vi "NI_9222_Anologue_DAQ3_FPGA_Host.vi"() -> ()   [LabVIEW 2013]
uses:
  <vilib>/userDefined/High Color/nirio_resource_hc.ctl
  <vilib>/rvi/interface/common/niFpgaWaitOnOcc.vi
  <vilib>/FPGAPlugInAG/cRIO-9068/niLvFpga_Open_cRIO-9068.vi
  <vilib>/rvi/interface/common/dynamic/niFpgaDynamicAddResources.vi
  <vilib>/Utility/error.llb/Error Cluster From Error Code.vi
  <vilib>/rvi/errors/niLvFpgaAdjustHostInterfaceError.vi
  <vilib>/RVI Host/nirviSupport.llb/nirviErrorClusterFromErrorCode.vi
  <vilib>/FPGAPlugInAG/Dynamic/niLvFpga_Close_Dynamic.vi
  <vilib>/rvi/interface/nirviOpenFPGA/nirviOpenFPGA.xnode
  FPGA Bitfiles/cRioProject1_FPGATarget_NI9222AnologueDA_7Q1sMVkmokY.lvbitx
  NI_9222_Anologue_DAQ2_FPGA.vi
  <vilib>/rvi/interface/nirviMethod/nirviMethod.xnode
  <vilib>/rvi/interface/nirviReadWriteControl/nirviReadWriteControl.xnode
  <vilib>/rvi/interface/nirviCloseFPGA/nirviCloseFPGA.xnode
  <vilib>/rvi/interface/Simulation/niFpgaSimulationCallBeginRW.vi
  NiFpgaLv.dll
  <vilib>/FPGAPlugInAG/Dynamic/niLvFpga_ReadFifo_Dynamic.vi
  <vilib>/rvi/errors/niLvFpgaMergeErrorWithErrorCode.vi
  <vilib>/rvi/interface/nirviMethod/StockFPGA_InlinedMethodWaitForSingleIRQ.vi
  <vilib>/FPGAPlugInAG/Dynamic/niLvFpga_WaitOnIrq_Dynamic.vi
  <vilib>/FPGAPlugInAG/Dynamic/niLvFpga_AcknowledgeIrq_Dynamic.vi
  <vilib>/FPGAPlugInAG/Dynamic/niLvFpga_StartFifo_Dynamic.vi
  <vilib>/FPGAPlugInAG/Dynamic/niLvFpga_ConfigureFifo_Dynamic.vi
panel:
  out "Array Out of FIFO size":i32[](array[numeric])
  out "time string":string
  out "Elements Remaining":u32
  out "FPGA Error Out 2":errorcluster
  in  "RIO Device":T1="RIO0"
  out "Timed Out":bool
  out "Sample Gated":bool
  out "Overwrite":bool
  in  "stop":bool
  out "FPGA Stop":bool
  out "Array to write size":i32[](array[numeric])
  out "Number of while loop iterations":i32
  in  "Sample Period (uSec)":u32=2
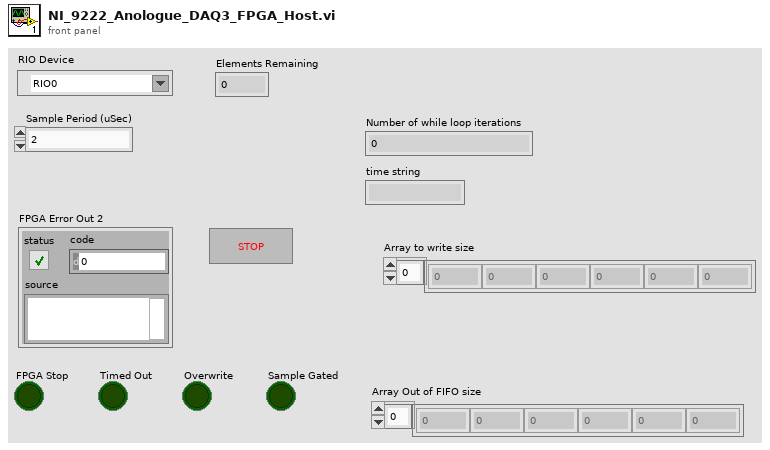
[diagram p1: front panel]
types:
  T1 = typedef "nirio_resource_hc.ctl" = tag
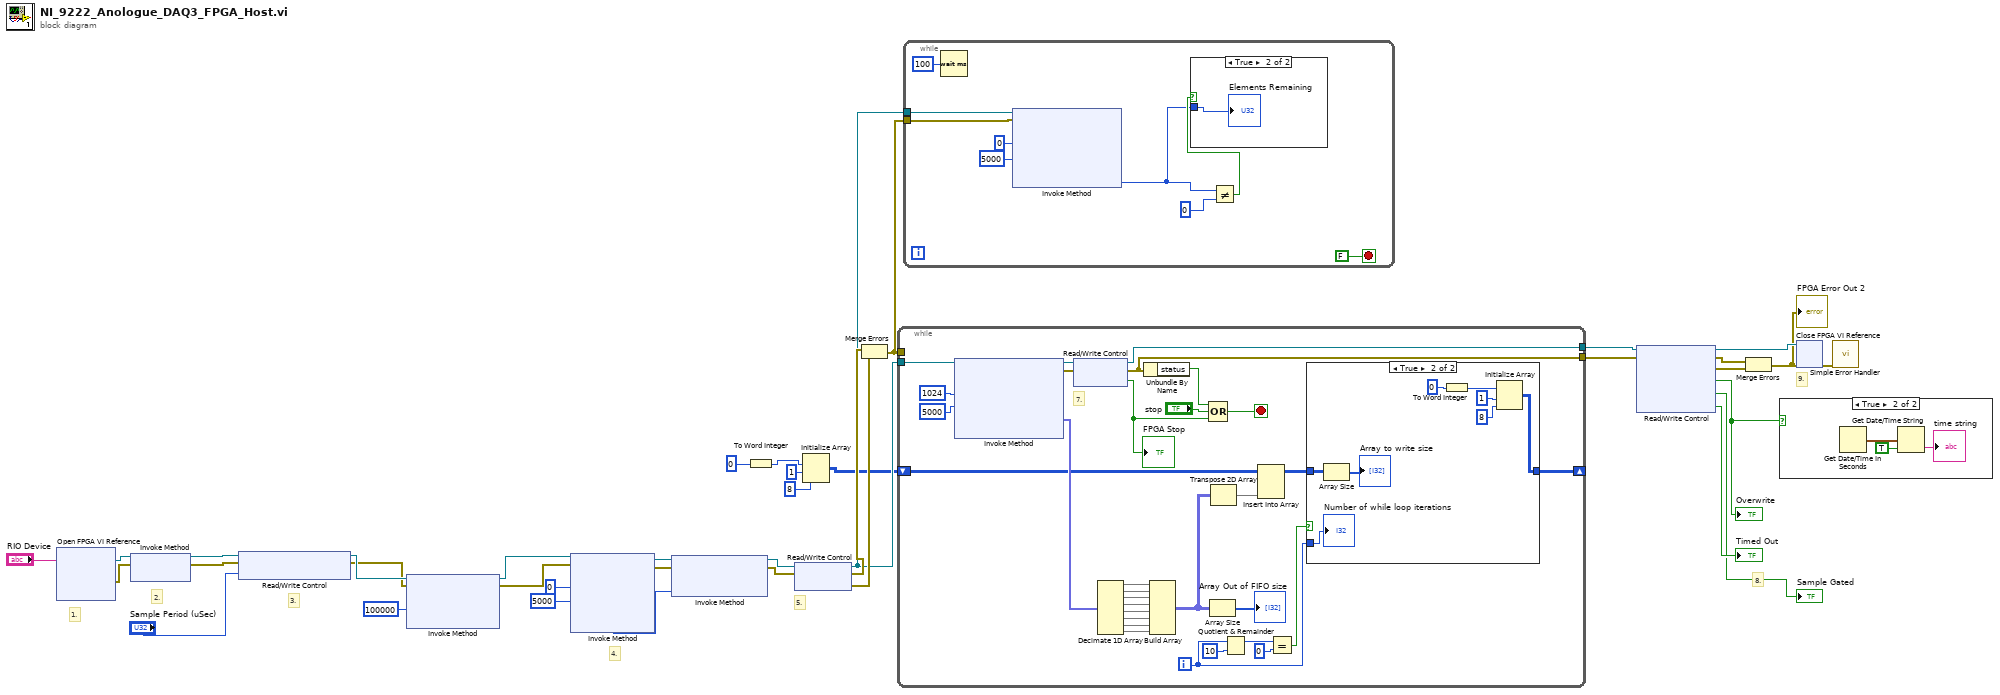
[diagram p0: block diagram]
diagram:
  # "5."
  # "4."
  # "9."
  # "8."
  # "3."
  # "2."
  # "1."
  n1 = xnode "Open FPGA VI Reference"("resource name"="RIO Device") -> ("FPGA VI Reference Out"=w35:refnum<k20>, "error out"=w36:errorcluster)  [unwired: 1 in]
  n2 = xnode "Invoke Method"("FPGA VI Reference In"=w35, "error in"=w36) -> ("FPGA VI Reference Out"=w34:refnum<k20>, "error out"=w33:errorcluster)
  n3 = xnode "Read/Write Control"("FPGA VI Reference In"=w34, "error in"=w33, "Sample Period (uSec)"="Sample Period (uSec)") -> ("FPGA VI Reference Out"=w5:refnum<k20>, "error out"=w3:errorcluster)
  n4 = xnode "Invoke Method"("FPGA VI Reference In"=w5, "error in"=w3, "Requested Depth"=u32 100000) -> ("FPGA VI Reference Out"=w4:refnum<k20>, "error out"=w2:errorcluster)  [unwired: 1 out]
  n5 = xnode "Invoke Method"("FPGA VI Reference In"=w4, "error in"=w2, "IRQ Number(s)"=0, "Timeout (ms)"=5000) -> ("FPGA VI Reference Out"=w20:refnum<k20>, "error out"=w21:errorcluster, "IRQ(s) Asserted"=w19:i32)  [unwired: 1 out]
  n6 = xnode "Invoke Method"("FPGA VI Reference In"=w20, "error in"=w21, "IRQ Number(s)"=w19) -> ("FPGA VI Reference Out"=w15:refnum<k20>, "error out"=w14:errorcluster)
  n7 = To Word Integer(number=i16 0) -> (16bit integer=w7:i16)
  n8 = xnode "Read/Write Control"("FPGA VI Reference In"=w15, "error in"=w14) -> ("FPGA VI Reference Out"=w13:refnum<k20>, "error out"=w23:errorcluster, "Error Out"=w22:errorcluster)
  n9 = Initialize Array(w7, 1 ("dimension size"), 8 ("dimension size")) -> (w10:i16[][])
  n10 = Merge Errors(w23, w22) -> (w12:errorcluster)
  n11 = while {
    tunnel: w13 -> [w47]
    tunnel: w12 -> [_]
    tunnel: [w67] -> w32
    tunnel: [w65] -> w31
    shift-right: [w58] -> _
    shift-left: w10 -> [w40]
    i -> [w57]
    stop <- w66 stop-if-true
    # "7."
    n12 = xnode "Invoke Method"("FPGA VI Reference In"=w47, "Number of Elements"=u32 1024, "Timeout (ms)"=5000) -> ("FPGA VI Reference Out"=w44:refnum<k20>, "error out"=w43:errorcluster, "Data"=w48:fxp<+/-,24,5>[])  [unwired: 1 in, 1 out]
    n13 = xnode "Read/Write Control"("FPGA VI Reference In"=w44, "error in"=w43) -> ("FPGA VI Reference Out"=w67:refnum<k20>, "error out"=w65:errorcluster, "Stopped"=w63:bool)
    "FPGA Stop" <- w63
    n14 = Decimate 1D Array(w48) -> (w52:fxp<+/-,24,5>[], w51:fxp<+/-,24,5>[], w50:fxp<+/-,24,5>[], w49:fxp<+/-,24,5>[], w53:fxp<+/-,24,5>[], w54:fxp<+/-,24,5>[], w55:fxp<+/-,24,5>[], w56:fxp<+/-,24,5>[])
    n15 = Unbundle By Name(w65) -> ("status"=w68:bool)
    n16 = Build Array(w52, w51, w50, w49, w53, w54, w55, w56) -> (w41:fxp<+/-,24,5>[][])
    n17 = Compound Arithmetic op=OR(w68, "stop", w63) -> (w66:bool)
    n18 = Array Size(array=w41) -> (size(s)=→"Array Out of FIFO size":i32[])
    n19 = Transpose 2D Array(2D array=w41) -> (transposed array=w38:fxp<+/-,24,5>[][])
    n20 = Quotient & Remainder(x=w57, y=10) -> (x-y*floor(x/y)=w61:i32)  [unwired: 1 out]
    n21 = Insert Into Array(array=w40, new element=w38) -> (w39:i16[][])  [unwired: 2 in]
    n22 = Equal?(x=w61, y=0) -> (x = y?=w59:bool)
    n23 = case shown="True" w59 {
      tunnel: w39 -> [w69 w77]
      tunnel: [w69 w71] -> w58
      tunnel: w57 -> [_ w76]
      frame False {
      }
      frame True {
        n24 = Array Size(array=w77) -> (size(s)=→"Array to write size":i32[])
        n25 = To Word Integer(number=i16 0) -> (16bit integer=w73:i16)
        n26 = Initialize Array(w73, 1 ("dimension size"), 8 ("dimension size")) -> (w71:i16[][])
        "Number of while loop iterations" <- w76
      }
    }
  }
  n27 = while {
    tunnel: w13 -> [w86]
    tunnel: w12 -> [w85]
    stop <- FALSE stop-if-true
    n28 = Wait (ms)(milliseconds to wait=u32 100) -> ()  [unwired: 1 out]
    n29 = xnode "Invoke Method"("FPGA VI Reference In"=w86, "error in"=w85, "Number of Elements"=u32 0, "Timeout (ms)"=5000) -> ("Elements Remaining"=w78:u32)  [unwired: 3 out]
    n30 = Not Equal?(x=w78, y=u32 0) -> (x != y?=w79:bool)
    n31 = case shown="True" w79 {
      tunnel: w78 -> [_ w87]
      frame False {
      }
      frame True {
        "Elements Remaining" <- w87
      }
    }
  }
  n32 = xnode "Read/Write Control"("FPGA VI Reference In"=w32, "error in"=w31) -> ("FPGA VI Reference Out"=w30:refnum<k20>, "error out"=w25:errorcluster, "Error Out"=w26:errorcluster, "Overwrite"=w11:bool, "Sample Gated"=→"Sample Gated":bool, "Timed Out"=→"Timed Out":bool)
  "Overwrite" <- w11
  n33 = Merge Errors(w25, w26) -> (w16:errorcluster)
  "FPGA Error Out 2" <- w16
  n34 = case shown="True" w11 {
    frame False {
    }
    frame True {
      n35 = Get Date/Time In Seconds() -> (seconds since 1Jan1904=w88:timestamp)
      n36 = Get Date/Time String(seconds (now)=w88, want seconds? (F)=TRUE) -> (time string=→"time string":string)  [unwired: 1 in, 1 out]
    }
  }
  n37 = xnode "Close FPGA VI Reference"("FPGA VI Reference In"=w30, "error in"=w16) -> ("error out"=w24:errorcluster)
  n38 = call <vilib>:"Simple Error Handler.vi"("error in (no error)"=w24) -> ()  [unwired: 4 in, 5 out]
